vi "TimerEngine.Update.vi"(8 "error in (no error)":errorcluster, 10 "TimePassed":i32, 11 "data value reference":refnum<data-value>) -> (0 "error out":errorcluster, 1 "Cache.TimePeroid(ms)":i32, 2 "Triggered":T1[](array[typedef]), 3 "data value reference 2":refnum<data-value>)   [LabVIEW 2017, in "TimerEngine.lvlib" / "TimerEngine.lvclass"]
uses:
  TimerEngine.lvclass
  _Typedef/Timer-UserEvent.ctl
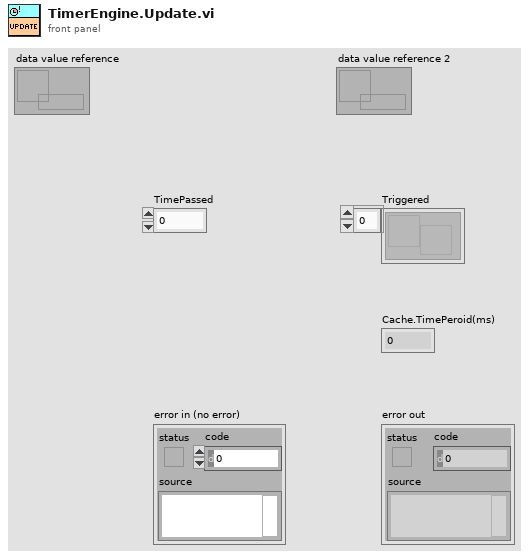
[diagram p1: front panel]
types:
  T1 = typedef "TimerEngine.lvlib/TimerEngine.lvclass/Timer-Userevent.ctl" = refnum<user-event>
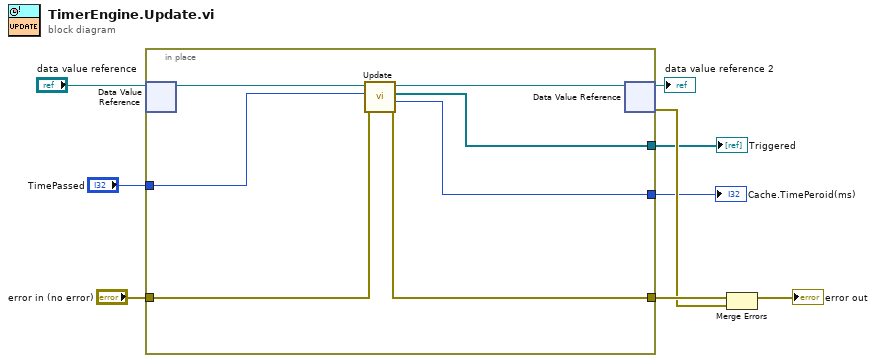
[diagram p0: block diagram]
diagram:
  n1 = in-place "In Place Element Structure" {
    in-place-border: [w10] -> w9
    in-place-border: "error in (no error)" -> [w11]
    in-place-border: [w14] -> w5
    in-place-border: [w13] -> w4
    in-place-border: "TimePassed" -> [w12]
    n2 = in-place-dvr #1("data value reference") -> (w16:refnum<class "TimerEngine.lvclass">)  [unwired: 1 out]
    n3 = call "Update.vi"("error in (no error)"=w11, "TimePassed"=w12, "UserEventTimer in"=w16) -> ("error out"=w10:errorcluster, "Cache.TimePeroid(ms)"=w13:i32, "Triggered"=w14:T1[], "UserEventTimer out"=w15:refnum<class "TimerEngine.lvclass">)  [unwired: 5 in]
    n4 = in-place-dvr #1(w15) -> (→"data value reference 2":refnum<data-value>, w6:errorcluster)
  }
  "Cache.TimePeroid(ms)" <- w4
  "Triggered" <- w5
  n5 = Merge Errors(w9, w6) -> (→"error out":errorcluster)
